vi "TAI_Solenoid.vi"(3 "Normal Output":bool, 4 "Aux Trigger":bool, 5 "Override Actuator Bypass":bool, 6 "Actuator Name":string) -> (0 "Interlocked Output":bool, 2 "Output Mode":T1(ring))   [LabVIEW 2020]
doc: "This VI is configured for polymorphic use and functions as an interlock, allowing the selected solenoid to be tested manually via the FRC 4265 Dashboard. During testing, all interlocked actuators which are not selected for testing are disabled."
uses:
  426a8fd3-0d55-4a18-942b-cc1f45a662fb.vi
  5c3c21bf-09c1-44ef-91a2-f0b618cdbb00.vi
  GlobalDriverStationData.vi
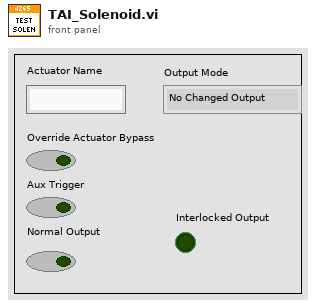
[diagram p1: front panel]
types:
  T1 = enum16{"No Changed Output", "New Normal Output", "New Testing Output"}
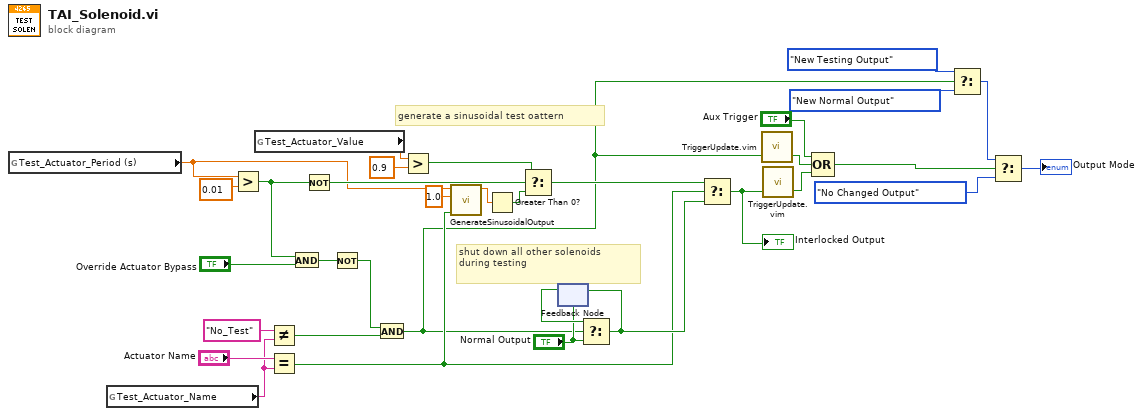
[diagram p0: block diagram]
diagram:
  # "generate a sinusoidal test oattern"
  # "shut down all other solenoids\nduring testing"
  n1 = global read "GlobalDriverStationData.vi" "Test_Actuator_Period (s)"() -> (w20:dbl)
  n2 = global read "GlobalDriverStationData.vi" "Test_Actuator_Name"() -> (w29:string)
  n3 = Greater?(x=w20, y=0.01) -> (0:w25:bool)
  n4 = global read "GlobalDriverStationData.vi" "Test_Actuator_Value"() -> (w21:dbl)
  n5 = Not Equal?(x="No_Test", y=w29) -> (x != y?=w13:bool)
  n6 = Equal?(x="Actuator Name", y=w29) -> (x = y?=w5:bool)
  n7 = And(x=w25, y="Override Actuator Bypass") -> (x .and. y?=w15:bool)
  n8 = Not(x=w25) -> (.not. x?=w24:bool)
  n9 = Not(x=w15) -> (.not. x?=w14:bool)
  n10 = And(x=w14, y=w13) -> (x .and. y?=w2:bool)
  n11 = Greater?(x=w21, y=0.9) -> (0:w22:bool)
  n12 = call "GenerateSinusoidalOutput.vi"("Init"=w5, "Amplitude"=1.0, "Period (s)"=w20) -> ("sin(time)"=w18:dbl)  [unwired: 8 in]
  n13 = Greater Than 0?(x=w18) -> (x > 0?=w17:bool)
  n14 = Select(t=w22, s=w24, f=w17) -> (s? t:f=w16:bool)
  n15 = feedback #1("Normal Output") -> (w30:bool)
  n16 = Select(t=w30, s=w2, f="Normal Output") -> (s? t:f=w31:bool)
  n17 = feedback-in #1(w31) -> ()
  n18 = Select(t=w16, s=w5, f=w31) -> (s? t:f=w7:bool)
  "Interlocked Output" <- w7
  n19 = call "TriggerUpdate.vim"("Trigger"=w2) -> ("Update"=w6:bool)  [unwired: 2 in]
  n20 = call "TriggerUpdate.vim"("Trigger"=w7) -> ("Update"=w4:bool)  [unwired: 2 in]
  n21 = Compound Arithmetic op=OR("Aux Trigger", w6, w4) -> (w3:bool)
  n22 = Select(t=T1."New Testing Output", s=w2, f=T1."New Normal Output") -> (s? t:f=w10:T1)
  n23 = Select(t=w10, s=w3, f=T1."No Changed Output") -> (s? t:f=→"Output Mode":T1)
